vi "Import Commands.vi"(8 "error in":errorcluster) -> (0 "error out":errorcluster, 3 "Imported Commands":string[][](array[string]))   [LabVIEW 2020]
uses:
  <vilib>/Utility/NIReport.llb/Report Type.ctl
  <vilib>/addons/_office/excel.llb/Excel Get Data ([str]).vi
  <vilib>/Utility/NIReport.llb/NI_report.lvclass
  <vilib>/addons/_office/NI_ReportGenerationToolkit.lvlib
  <vilib>/Utility/NIReport.llb/NI_ReportGenerationCore.lvlib
  <vilib>/Utility/NIReport.llb/Excel/NI_Excel.lvclass
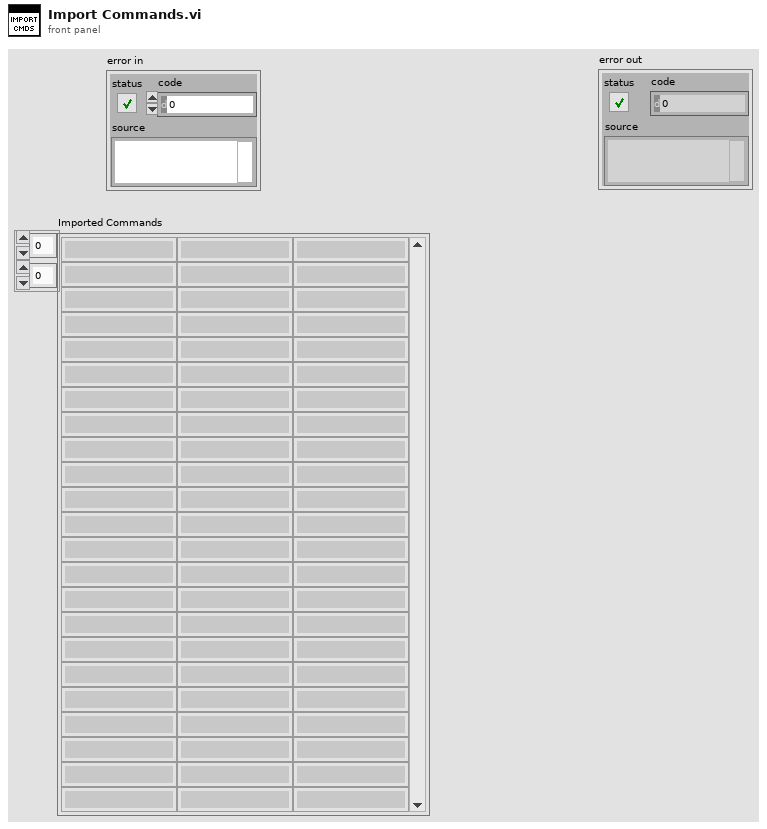
[diagram p1: front panel]
types:
  T1 = typedef "NI_ReportGenerationCore.lvlib/Report Type.ctl" = enum16{"HTML", "Word", "Excel"}
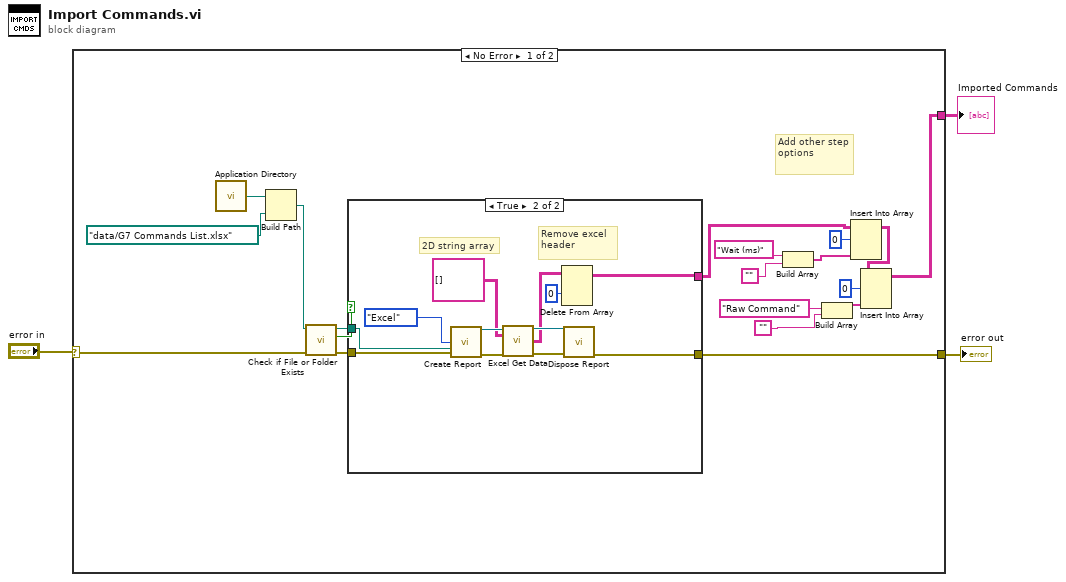
[diagram p0: block diagram]
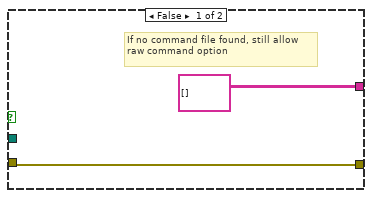
[diagram p2: hidden frame]
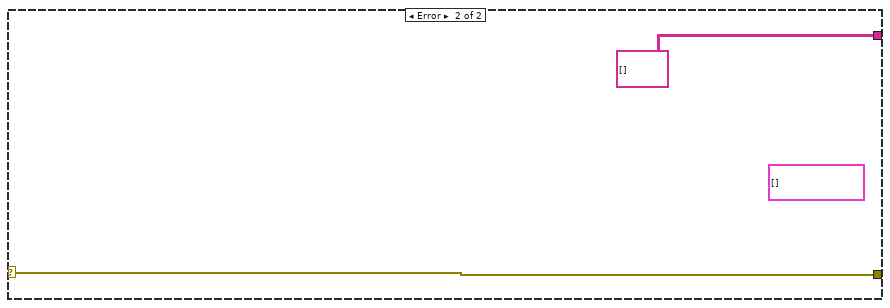
[diagram p3: hidden frame]
diagram:
  n1 = case shown="No Error" "error in" {
    selector: "error in" -> [w20 w38]
    tunnel: [w18 w38] -> w2
    tunnel: [w14 string[][] [] ("data")] -> w1
    frame No Error {
      # "Add other step options"
      n2 = call <vilib>:"Application Directory.vi"() -> ("Application Directory"=w13:path)
      n3 = Build Path(base path=w13, name or relative path=path "data/G7 Commands List.xlsx" ("Path")) -> (appended path=w11:path)
      n4 = call <vilib>:"Check if File or Folder Exists.vi"("error in (no error)"=w20, "path"=w11) -> ("error out"=w19:errorcluster, "file or folder exists?"=w22:bool, "dup path"=w21:path)  [unwired: 7 in]
      n5 = case shown="True" w22 {
        tunnel: [string[][] [] ("data") w25] -> w5
        tunnel: w21 -> [_ w35]
        tunnel: w19 -> [w23 w34]
        tunnel: [w23 w33] -> w18
        frame False {
          # "If no command file found, still allow raw command option"
        }
        frame True {
          # "Remove excel header"
          # "2D string array"
          n6 = call <vilib>:"Create Report.vi"("report type"=Report_Type."Excel", "template (empty)"=w35, "error in (no error)"=w34) -> ("report out"=w32:refnum<class "NI_report.lvclass">, "error out"=w30:errorcluster)  [unwired: 11 in]
          n7 = call-poly <vilib>:"Excel Get Data.vi"("report in"=w32, "data type"=string[][] [], "error in (no error)"=w30) -> ("report out"=w31:refnum<class "NI_report.lvclass">, "data"=w27:string[][], "error out"=w29:errorcluster)  [unwired: 10 in]
          n8 = Delete From Array(array=w27, index (row)=0) -> (array with subset deleted=w25:string[][])  [unwired: 2 in, 1 out]
          n9 = call-dynamic "Dispose Report.vi"("report in"=w31, "error in (no error)"=w29) -> ("error out"=w33:errorcluster)  [unwired: 13 in]
        }
      }
      n10 = Build Array("Wait (ms)", "") -> (w6:string[])
      n11 = Build Array("Raw Command", "") -> (w17:string[])
      n12 = Insert Into Array(array=w5, index (row)=0, new element=w6) -> (w4:string[][])  [unwired: 1 in]
      n13 = Insert Into Array(array=w4, index (row)=0, new element=w17) -> (w14:string[][])  [unwired: 1 in]
    }
    frame Error {
      (unwired) cluster{"data":string[]}[] []
    }
  }
  "error out" <- w2
  "Imported Commands" <- w1
